vi "Write Single Holding Register.vi"(7 "unit ID":u8, 8 "error in":errorcluster, 9 "register to write":u16, 10 "address":u16, 11 "Modbus master in":refnum<class "Modbus Master.lvclass">) -> (0 "error out":errorcluster, 3 "Modbus master out":refnum<class "Modbus Master.lvclass">)   [LabVIEW 2013, in "Modbus Library - Advance.lvlib" / "Modbus Master.lvclass"]
doc: "Writes <B>register to write</B> to <B>address</B> of the device."
uses:
  Modbus Master.lvclass
  Modbus Master.lvclass/Modbus Master.ctl
  Modbus API.lvclass/Modbus API.ctl
  Transmission Data Unit/Transmission Data Unit.lvclass/Transmission Data Unit.ctl
  Transmission Data Unit/Transmission Data Unit.lvclass
  Master Function Definition/Master Function Definition.lvclass
  Modbus API.lvclass
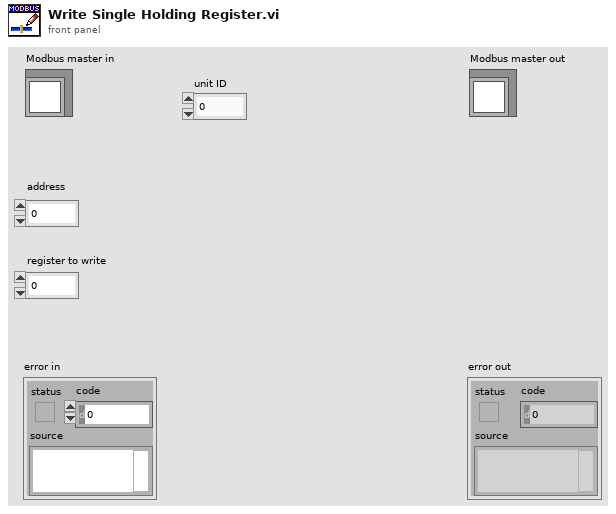
[diagram p1: front panel]
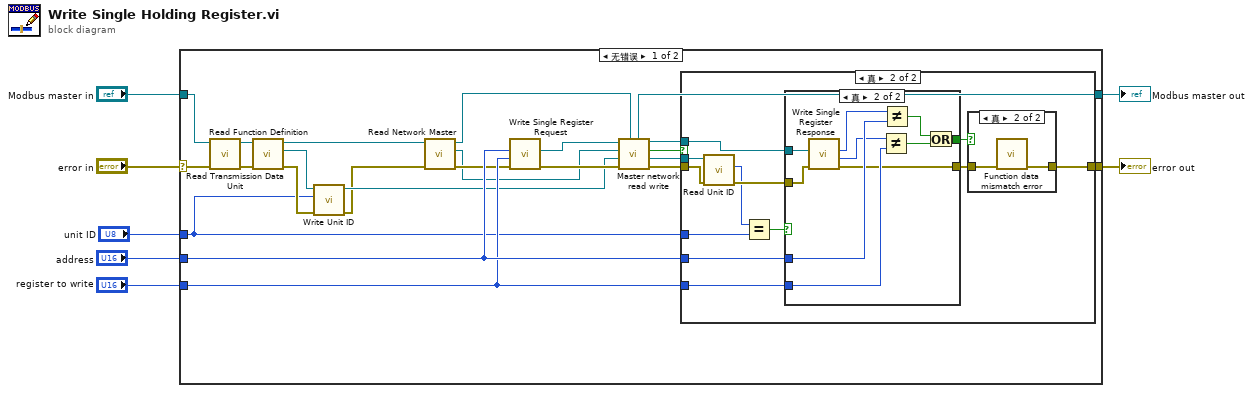
[diagram p0: block diagram]
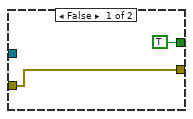
[diagram p3: hidden frame]
diagram:
  n1 = case shown="无错误" "error in" {
    selector: "error in" -> [w19 w59]
    tunnel: "Modbus master in" -> [w17 w60]
    tunnel: [w23 w60] -> w5
    tunnel: [w29 w59] -> w4
    tunnel: "address" -> [w28 _]
    tunnel: "register to write" -> [w27 _]
    tunnel: "unit ID" -> [w9 _]
    frame No Error {
      n2 = call "Read Function Definition.vi"("error in"=w19, "Modbus master in"=w17) -> ("error out"=w21:errorcluster, "Modbus master out"=w20:refnum<class "Modbus Master.lvclass">)  [unwired: 7 in, 1 out]
      n3 = call "Read Transmission Data Unit.vi"("error in"=w21, "Modbus instance in"=w20) -> ("error out"=w11:errorcluster, "transmission data unit"=w13:refnum<class "Transmission Data Unit.lvclass">, "Modbus instance out"=w22:refnum<class "Modbus Master.lvclass">)  [unwired: 7 in]
      n4 = call "Write Unit ID.vi"("error in"=w11, "unit ID"=w9, "transmission data unit in"=w13) -> ("error out"=w10:errorcluster, "transmission data unit out"=w12:refnum<class "Transmission Data Unit.lvclass">)  [unwired: 7 in]
      n5 = call "Read Network Master.vi"("error in"=w10, "Modbus master in"=w22) -> ("error out"=w18:errorcluster, "network master"=w15:refnum<class "Network Master.lvclass">, "Modbus master out"=w16:refnum<class "Modbus Master.lvclass">)  [unwired: 7 in]
      n6 = call "Write Single Register Request.vi"("error in"=w18, "Register Value"=w27, "Starting Address"=w28) -> ("error out"=w30:errorcluster, "modbus data unit out"=w25:refnum<class "Modbus Data Unit.lvclass">)  [unwired: 7 in]
      n7 = call "Master network read write.vi"("Modbus master in"=w16, "error in"=w30, "transmission data unit in"=w12, "network master in"=w15, "Modbus data unit in"=w25) -> ("error out"=w26:errorcluster, "transmission data unit out"=w8:refnum<class "Transmission Data Unit.lvclass">, "PDU Valid?"=w14:bool, "Modbus data unit out"=w24:refnum<class "Modbus Data Unit.lvclass">, "Modbus master out"=w23:refnum<class "Modbus Master.lvclass">)  [unwired: 2 in]
      n8 = case shown="真" w14 {
        tunnel: [w31 w42] -> w29
        tunnel: w28 -> [_ w41]
        tunnel: w27 -> [_ w40]
        tunnel: w26 -> [w31 w36]
        tunnel: w24 -> [_ w39]
        tunnel: w9 -> [_ w33]
        tunnel: w8 -> [_ w37]
        frame False {
        }
        frame True {
          n9 = call "Read Unit ID.vi"("error in"=w36, "transmission data unit in"=w37) -> ("error out"=w35:errorcluster, "unit ID"=w34:u8)  [unwired: 7 in, 1 out]
          n10 = Equal?(x=w34, y=w33) -> (x = y?=w32:bool)
          n11 = case shown="真" w32 {
            tunnel: [TRUE w53] -> w43
            tunnel: w41 -> [_ w51]
            tunnel: w40 -> [_ w50]
            tunnel: w39 -> [_ w48]
            tunnel: [w45 w47] -> w38
            tunnel: w35 -> [w45 w46]
            frame False {
            }
            frame True {
              n12 = call "Write Single Register Response.vi"("error in"=w46, "modbus data unit in"=w48) -> ("error out"=w47:errorcluster, "Number of Coils"=w49:u16, "Address"=w52:u16)  [unwired: 7 in]
              n13 = Not Equal?(x=w49, y=w50) -> (x != y?=w55:bool)
              n14 = Not Equal?(x=w52, y=w51) -> (x != y?=w54:bool)
              n15 = Or(x=w54, y=w55) -> (x .or. y?=w53:bool)
            }
          }
          n16 = case shown="真" w43 {
            tunnel: [w56 w58] -> w42
            tunnel: w38 -> [w56 w57]
            frame False {
            }
            frame True {
              n17 = call "Function data mismatch error.vi"("error in (no error)"=w57) -> ("error out"=w58:errorcluster)  [unwired: 10 in]
            }
          }
        }
      }
    }
    frame Error {
    }
  }
  "error out" <- w4
  "Modbus master out" <- w5
